vi "Shift Register Delay.vi"(9 "input":dbl, 10 "n delay(0)":i32) -> (2 "output":dbl)   [LabVIEW 2010]
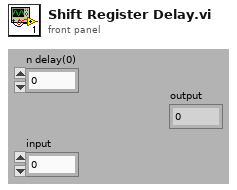
[diagram p1: front panel]
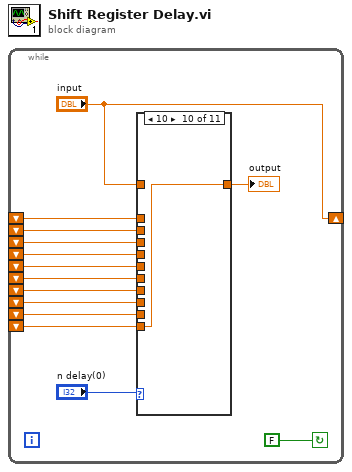
[diagram p0: block diagram]
diagram:
  n1 = while {
    shift-right: ["input"] -> _
    shift-left: _ -> [w10]
    shift-left: _ -> [w9]
    shift-left: _ -> [w8]
    shift-left: _ -> [w7]
    shift-left: _ -> [w6]
    shift-left: _ -> [w5]
    shift-left: _ -> [w4]
    shift-left: _ -> [w3]
    shift-left: _ -> [w2]
    shift-left: _ -> [w1]
    stop <- FALSE continue-if-true
    n2 = case shown="10" "n delay(0)" {
      tunnel: "input" -> [_ _ _ _ _ _ _ _ _ _ w25]
      tunnel: [w15 w16 w17 w18 w19 w20 w21 w22 w23 w24 w25] -> w12
      tunnel: w10 -> [w15 _ _ _ _ _ _ _ _ _ _]
      tunnel: w9 -> [_ w16 _ _ _ _ _ _ _ _ _]
      tunnel: w8 -> [_ _ w17 _ _ _ _ _ _ _ _]
      tunnel: w7 -> [_ _ _ w18 _ _ _ _ _ _ _]
      tunnel: w6 -> [_ _ _ _ w19 _ _ _ _ _ _]
      tunnel: w5 -> [_ _ _ _ _ w20 _ _ _ _ _]
      tunnel: w4 -> [_ _ _ _ _ _ w21 _ _ _ _]
      tunnel: w3 -> [_ _ _ _ _ _ _ w22 _ _ _]
      tunnel: w2 -> [_ _ _ _ _ _ _ _ w23 _ _]
      tunnel: w1 -> [_ _ _ _ _ _ _ _ _ w24 _]
      frame 1 {
      }
      frame 2 {
      }
      frame 3 {
      }
      frame 4 {
      }
      frame 5 {
      }
      frame 6 {
      }
      frame 7 {
      }
      frame 8 {
      }
      frame 9 {
      }
      frame 10 {
      }
      frame 0, Default {
      }
    }
    "output" <- w12
  }
